vi "Channel Probe.vi"(2 "channelOp":T2(ring), 3 "mdata in":refnum<class "MessengerMBase.lvclass">) -> (1 "mdata out":refnum<class "MessengerMBase.lvclass">)   [LabVIEW 2019, in "MessengerM.lvlib"]
doc: "Displays the status of the channel as the channel is modified by the various endpoints and gives the user ways to pause the application using the channel."
uses:
  <resource>/Channels/MessengerM/MessengerM.lvlib
  <resource>/Channels/MessengerM/MessengerMBase/MessengerMBase.lvclass
  <resource>/Channels/MessengerM/Element.ctl
panel:
  out "GUID":string
  out "Active?":bool
  in  "subchannel":i32
  out "elements":cluster{"elt":T1}[](array[cluster])
  in  "Message ID to match":u32
  in  "Details":string="Details"
  in  "Latest Message ID":string="Latest Message ID:"
  out "Details":string
  in  "Last Operation":string="Last Operation:"
  in  "Read":string="Read"
  in  "Write":string="Write"
  in  "Single Step":bool
  in  "Pause when latest message ID matches":bool
  in  "Pause when aborted":bool
  in  "Pause when any last element written":bool
  in  "Fixed Size":string="<b>Current Element Count:</b>\n%d\n<b>Allocated Element Count:</b>\n%d (Fixed Size)\n"
  out "Details":string
  in  "Play":bool
  out "Aborted?":bool
  out "Last element written?":bool
  in  "Pause":bool
  out "No Endpoiont Yet":string="\n\n\n\n\n\n\n\n\n\n\nNeither endpoint has executed yet."
  in  "Message Index":i32 min=0
  in  "Unbounded":string="<b>Current Element Count:</b>\n%d\n<b>Allocated Element Count:</b>\n%d (Unbounded)\n"
  out "Latest":string="Latest\nEnqueue"
  out "Next":string="Next\nDequeue"
  # "Details"
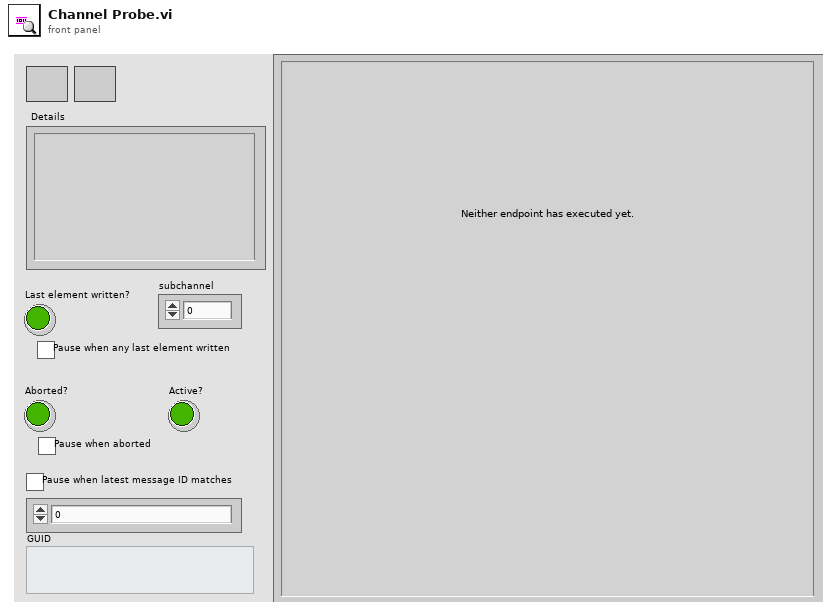
[diagram p1: front panel]
types:
  T1 = typedef "MessengerM.lvlib/Element.ctl" = string
  T2 = enum16{"init", "write", "read", "wrtAck", "rdAck", "rdAck2", "probe"}
  T3 = enum32{"Invalid", "Standard", "Closed", "Hidden", "Minimized", "Maximized"}
  T4 = cluster{"count":i32, "size":i32, "array":cluster{"elt":T1}[], "unbounded":bool, "active":bool, "last elt":bool, "GUID":string}[]
  T5 = cluster{"count":i32, "size":i32, "array":cluster{"elt":T1}[], "unbounded":bool, "active":bool, "last elt":bool, "GUID":string}
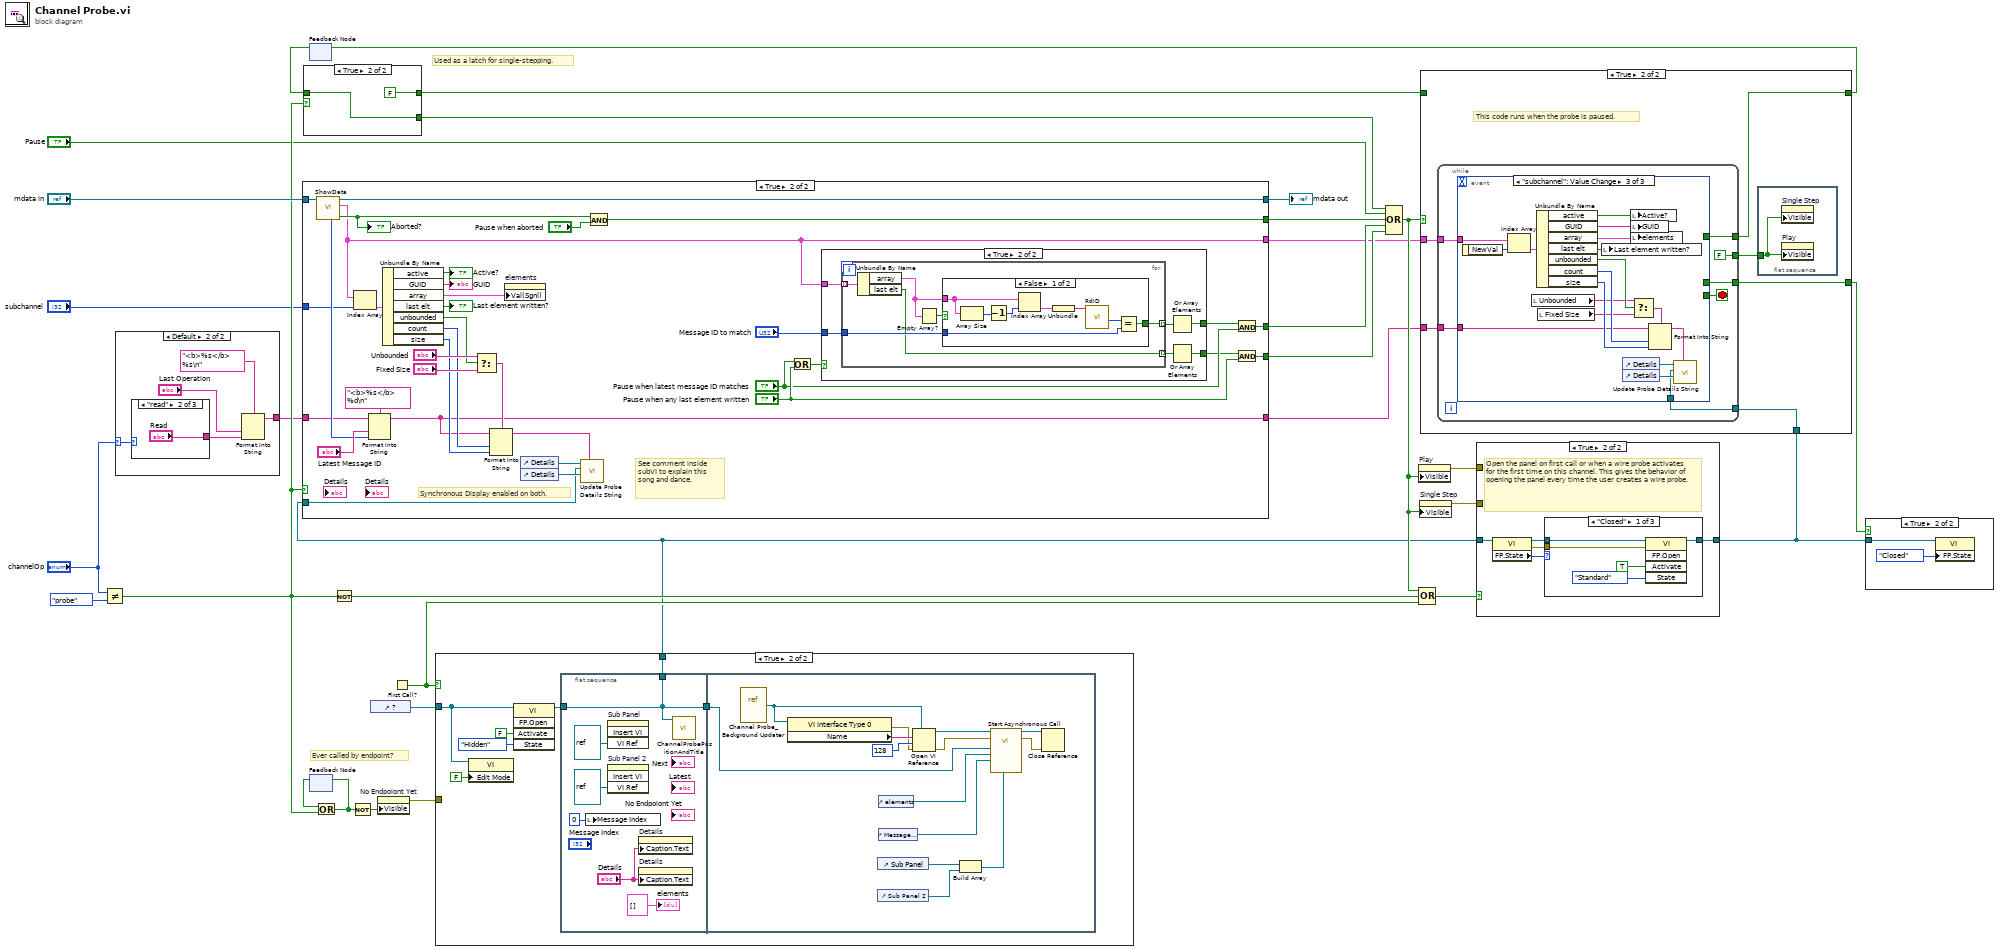
[diagram p0: block diagram]
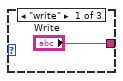
[diagram p3: hidden frame]
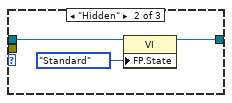
[diagram p11: hidden frame]
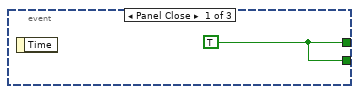
[diagram p14: hidden frame]
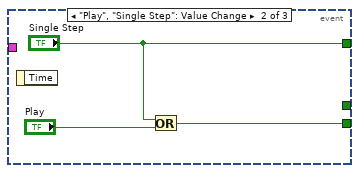
[diagram p15: hidden frame]
diagram:
  # "Used as a latch for single-stepping."
  # "Ever called by endpoint?"
  n1 = Not Equal?(x="channelOp", y=T2."probe" ("channelOp")) -> (x != y?=w13:bool)
  n2 = case shown="Default" "channelOp" {
    selector: "channelOp" -> [_ w36]
    tunnel: [_ w34] -> w9
    frame "init", "probe" {
    }
    frame Default {
      n3 = case shown="\"read\"" w36 {
        tunnel: ["Write" "Read" _] -> w33
        frame "write" {
        }
        frame "read" {
        }
        frame Default {
        }
      }
      n4 = Format Into String(format string="<b>%s</b> %s\n", "Last Operation", w33) -> (resulting string=w34:string)  [unwired: 2 in, 1 out]
    }
  }
  n5 = feedback #1() -> (w19:bool)  [unwired: 1 in]
  n6 = case shown="True" w13 {
    tunnel: w19 -> [w39 w40]
    tunnel: [w39 FALSE] -> w18
    tunnel: [_ w40] -> w17
    frame False {
    }
    frame True {
    }
  }
  n7 = feedback #2() -> (w25:bool)  [unwired: 1 in]
  n8 = Or(x=w25, y=w13) -> (x .or. y?=w24:bool)
  n9 = feedback-in #2(w24) -> ()
  n10 = Not(x=w13) -> (.not. x?=w12:bool)
  n11 = Not(x=w24) -> (.not. x?=w21:bool)
  n12 = control-ref of="?"() -> (w26:refnum<vi>)
  n13 = property on="No Endpoiont Yet" class="Str"("Visible"=w21) -> (error out=w23:errorcluster)  [unwired: 2 in, 1 out]
  n14 = First Call?() -> (First Call?: T/F=w11:bool)
  n15 = case shown="True" w11 {
    tunnel: [w42 w49] -> w3
    tunnel: w26 -> [w42 w43]
    tunnel: w23 -> [_ _]
    frame False {
    }
    frame True {
      n16 = property class="VI"(reference=w43, "Edit Mode"=FALSE ("Edit Mode On Open")) -> ()  [unwired: 1 in, 2 out]
      n17 = invoke class="VI" method="FP.Open"(reference=w43, "Activate"=FALSE ("Activate?"), "State"=T3."Hidden") -> (reference out=w46:refnum<vi>)  [unwired: 2 in, 4 out]
      n18 = flat-sequence {
        tunnel: [w51] -> w49
        tunnel: w46 -> [w51]
        tunnel: [w51] -> w44
        tunnel: w44 -> [w58]
        frame #0 {
          n19 = local write "Message Index"(0 ("Message Index")) -> ()
          n20 = invoke on="Sub Panel" class="SubPnl" method="Insert VI"("VI Ref"=refnum<vi> refnum) -> ()  [unwired: 3 in, 4 out]
          n21 = invoke on="Sub Panel 2" class="SubPnl" method="Insert VI"("VI Ref"=refnum<vi> refnum) -> ()  [unwired: 3 in, 4 out]
          n22 = property on="Details" class="Str"("Caption.Text"="Details") -> ()  [unwired: 2 in, 2 out]
          n23 = property on="Details" class="Str"("Caption.Text"="Details") -> ()  [unwired: 2 in, 2 out]
          n24 = call <resource>:"ChannelProbePositionAndTitle.vi"("VI in"=w51) -> ()  [unwired: 9 in, 2 out]
          "elements" <- cluster{"elt":T1}[] [] ("elements")
        }
        frame #1 {
          n25 = vi-ref <resource>:"Channel Probe_Background Updater.vi"() -> (w68:refnum<vi>)
          n26 = property class="VI Interface Type 0"(reference=w68) -> (error out=w59:errorcluster, "Name"=w69:string)  [unwired: 1 in, 1 out]
          n27 = control-ref of="Sub Panel"() -> (w63:refnum<vi>)
          n28 = control-ref of="Sub Panel 2"() -> (w62:refnum<vi>)
          n29 = control-ref of="elements"() -> (w60:refnum<vi>)
          n30 = control-ref of="Message Index"() -> (w64:refnum<vi>)
          n31 = Open VI Reference(type specifier VI Refnum (for type only)=w68, vi path=w69, options=128, error in (no error)=w59) -> (vi reference=w66:refnum<vi>, error out=w65:errorcluster)  [unwired: 2 in]
          n32 = Build Array(w63, w62) -> (w61:refnum<vi>[])
          n33 = call-by-ref "Start Asynchronous Call"(reference=w66, error in=w65, "Subpanels"=w61, "Message Index ref"=w64, "elements"=w60, "VI Ref"=w58) -> (reference out=w56:refnum<vi>, error out=w57:errorcluster)  [unwired: 8 in]
          n34 = Close Reference(reference=w56, error in (no error)=w57) -> ()  [unwired: 1 out]
        }
      }
    }
  }
  n35 = case shown="True" w13 {
    tunnel: "mdata in" -> [w70 w94]
    tunnel: [_ w101] -> w29
    tunnel: [_ w80] -> w28
    tunnel: [_ w100] -> w27
    tunnel: w3 -> [_ w98]
    tunnel: w9 -> [_ w86]
    tunnel: [w70 w93] -> w8
    tunnel: "subchannel" -> [_ w88]
    tunnel: [_ w73] -> w2
    tunnel: [_ w71] -> w1
    frame False {
    }
    frame True {
      # "See comment inside subVI to explain this song and dance."
      # "Synchronous Display enabled on both."
      n36 = call-dynamic "ShowData.vi"("messengerMbase in"=w94) -> ("abort"=w91:bool, "subchannels"=w73:T4, "messengerMbase out"=w93:refnum<class "MessengerMBase.lvclass">, "lastID"=w92:u32)  [unwired: 6 in, 1 out]
      "Aborted?" <- w91
      n37 = Index Array(array=w73, index=w88) -> (element=w90:T5)
      n38 = Format Into String(format string="<b>%s</b> %d\n", initial string=w86, "Latest Message ID", w92) -> (resulting string=w71:string)  [unwired: 1 in, 1 out]
      n39 = Unbundle By Name(w90) -> ("active"=→"Active?":bool, "GUID"=→"GUID":string, "array"=w81:cluster{"elt":T1}[], "last elt"=→"Last element written?":bool, "unbounded"=w72:bool, "count"=w84:i32, "size"=w83:i32)
      n40 = Select(t="Unbounded", s=w72, f="Fixed Size") -> (s? t:f=w103:string)
      n41 = Format Into String(format string=w103, initial string=w71, w84, w83) -> (resulting string=w85:string)  [unwired: 1 in, 1 out]
      n42 = property on="elements" class="Arr (strict)"("Val(Sgnl)"=w81) -> ()  [unwired: 2 in, 2 out]
      n43 = control-ref of="Details"() -> (w97:refnum<vi>)
      n44 = control-ref of="Details"() -> (w99:refnum<vi>)
      n45 = call <resource>:"Update Probe Details String.vi"("String"=w85, "Details 1"=w99, "VI Reference"=w98, "Details 2"=w97) -> ()  [unwired: 8 in]
      n46 = And(x=w91, y="Pause when aborted") -> (x .and. y?=w101:bool)
      n47 = Or(x="Pause when latest message ID matches", y="Pause when any last element written") -> (x .or. y?=w78:bool)
      n48 = case shown="True" w78 {
        tunnel: w73 -> [_ w111]
        tunnel: "Message ID to match" -> [_ w110]
        tunnel: [_ w107] -> w76
        tunnel: [_ w106] -> w74
        frame False {
        }
        frame True {
          n49 = for {
            tunnel: [w117] -> w109 mode=indexing
            tunnel: w111 -> [w115] mode=indexing
            tunnel: w110 -> [w113]
            tunnel: [w112] -> w108 mode=indexing
            n50 = Unbundle By Name(w115) -> ("array"=w114:cluster{"elt":T1}[], "last elt"=w112:bool)
            n51 = Empty Array?(array=w114) -> (empty?=w116:bool)
            n52 = case shown="False" w116 {
              tunnel: [w123 _] -> w117
              tunnel: w114 -> [w122 _]
              tunnel: w113 -> [w118 _]
              frame False {
                n53 = Array Size(array=w122) -> (size(s)=w125:i32)
                n54 = Decrement(x=w125) -> (x-1=w124:i32)
                n55 = Index Array(array=w122, index=w124) -> (element=w121:cluster{"elt":T1})
                n56 = Unbundle(w121) -> ("elt"=w119:T1)
                n57 = call <resource>:"RdID.vi"("element in"=w119) -> ("id"=w120:u32)  [unwired: 10 in]
                n58 = Equal?(x=w120, y=w118) -> (x = y?=w123:bool)
              }
              frame True {
              }
            }
          }
          n59 = Or Array Elements(Boolean array=w109) -> (logical OR=w107:bool)
          n60 = Or Array Elements(Boolean array=w108) -> (logical OR=w106:bool)
        }
      }
      n61 = And(x=w76, y="Pause when latest message ID matches") -> (x .and. y?=w80:bool)
      n62 = And(x=w74, y="Pause when any last element written") -> (x .and. y?=w100:bool)
    }
  }
  "mdata out" <- w8
  n63 = Compound Arithmetic op=OR(w17, "Pause", w29, w28, w27) -> (w7:bool)
  n64 = property on="Play" class="Bool"("Visible"=w7) -> (error out=w15:errorcluster)  [unwired: 2 in, 1 out]
  n65 = Compound Arithmetic op=OR(w7, w12, w11) -> (w10:bool)
  n66 = property on="Single Step" class="Bool"("Visible"=w7) -> (error out=w16:errorcluster)  [unwired: 2 in, 1 out]
  n67 = case shown="True" w10 {
    tunnel: [w126 w128] -> w22
    tunnel: w3 -> [w126 w127]
    tunnel: w16 -> [_ _]
    tunnel: w15 -> [_ _]
    frame False {
    }
    frame True {
      # "Open the panel on first call or when a wire probe activates for the first time on this channel. This gives the behavior of opening the panel every time the user creates a wire probe."
      n68 = property class="VI"(reference=w127) -> (reference out=w129:refnum<vi>, error out=w130:errorcluster, "FP.State"=w131:T3)  [unwired: 1 in]
      n69 = case shown="\"Closed\"" w131 {
        tunnel: w130 -> [w135 _ _]
        tunnel: w129 -> [w136 w139 w140]
        tunnel: [w132 w138 w140] -> w128
        frame "Closed" {
          n70 = invoke class="VI" method="FP.Open"(reference=w136, error in=w135, "Activate"=TRUE ("Activate?"), "State"=T3."Standard") -> (reference out=w132:refnum<vi>)  [unwired: 1 in, 4 out]
        }
        frame "Hidden" {
          n71 = property class="VI"(reference=w139, "FP.State"=T3."Standard" ("Front Panel Window:State")) -> (reference out=w138:refnum<vi>)  [unwired: 1 in, 1 out]
        }
        frame Default {
        }
      }
    }
  }
  n72 = case shown="True" w7 {
    tunnel: w22 -> [_ w143]
    tunnel: [_ w147] -> w31
    tunnel: [w141 w145] -> w20
    tunnel: w18 -> [w141 _]
    tunnel: w2 -> [_ w144]
    tunnel: w1 -> [_ w142]
    frame False {
    }
    frame True {
      # "This code runs when the probe is paused."
      n73 = while {
        tunnel: [w155] -> w147
        tunnel: [FALSE ("Visible")] -> w146
        tunnel: [w152] -> w145
        tunnel: w144 -> [w151]
        tunnel: w143 -> [w150]
        tunnel: w142 -> [w149]
        stop <- w154 stop-if-true
        n74 = event shown="[2] \"subchannel\": Value Change" {
          selector: _ -> [_ _ _]
          dyn-events: _ -> [_ _ _]
          timeout: _ -> [_ _ _]
          tunnel: [w156 _ _] -> w155
          tunnel: [w156 w158 _] -> w154
          tunnel: [_ "Single Step" _] -> w152
          tunnel: w151 -> [_ _ w176]
          tunnel: w150 -> [_ _ w168]
          tunnel: w149 -> [_ _ w160]
          event Panel Close {
            w156 = TRUE
            n75 = event-data() -> ()  [unwired: 1 in, 1 out]
          }
          event "Play", "Single Step": Value Change {
            n76 = event-data() -> ()  [unwired: 1 in, 1 out]
            n77 = Or(x="Single Step", y="Play") -> (x .or. y?=w158:bool)
          }
          event "subchannel": Value Change {
            n78 = event-data() -> ("NewVal"=w175:i32)  [unwired: 1 in]
            n79 = Index Array(array=w176, index=w175) -> (element=w177:T5)
            n80 = local read "Unbounded"() -> (w162:string)
            n81 = Unbundle By Name(w177) -> ("active"=w174:bool, "GUID"=w173:string, "array"=w172:cluster{"elt":T1}[], "last elt"=w165:bool, "unbounded"=w164:bool, "count"=w166:i32, "size"=w167:i32)
            n82 = local read "Fixed Size"() -> (w161:string)
            n83 = local write "Last element written?"(w165) -> ()
            n84 = control-ref of="Details"() -> (w171:refnum<vi>)
            n85 = control-ref of="Details"() -> (w170:refnum<vi>)
            n86 = local write "Active?"(w174) -> ()
            n87 = local write "GUID"(w173) -> ()
            n88 = local write "elements"(w172) -> ()
            n89 = Select(t=w162, s=w164, f=w161) -> (s? t:f=w163:string)
            n90 = Format Into String(format string=w163, initial string=w160, w166, w167) -> (resulting string=w169:string)  [unwired: 1 in, 1 out]
            n91 = call <resource>:"Update Probe Details String.vi"("String"=w169, "Details 1"=w170, "VI Reference"=w168, "Details 2"=w171) -> ()  [unwired: 8 in]
          }
        }
      }
      n92 = flat-sequence {
        tunnel: w146 -> [w148]
        frame #0 {
          n93 = property on="Single Step" class="Bool"("Visible"=w148) -> ()  [unwired: 2 in, 2 out]
          n94 = property on="Play" class="Bool"("Visible"=w148) -> ()  [unwired: 2 in, 2 out]
        }
      }
    }
  }
  n95 = feedback-in #1(w20) -> ()
  n96 = case shown="True" w31 {
    tunnel: w22 -> [_ w178]
    frame False {
    }
    frame True {
      n97 = property class="VI"(reference=w178, "FP.State"=T3."Closed" ("Front Panel Window:State")) -> ()  [unwired: 1 in, 2 out]
    }
  }
